vi "Read Coins Config.vi"(8 "error in (no error)":errorcluster) -> (0 "error out":errorcluster, 3 "Value":cluster{"Bolean text":string, "Value":i32}[](array[cluster]))   [LabVIEW 2019, in "Monedas.lvlib"]
uses:
  Monedas.lvlib
  <vilib>/Utility/xml.llb/Read From XML File(string).vi
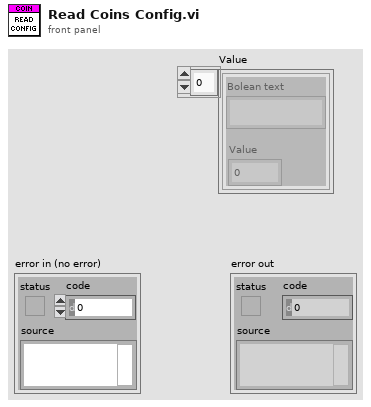
[diagram p1: front panel]
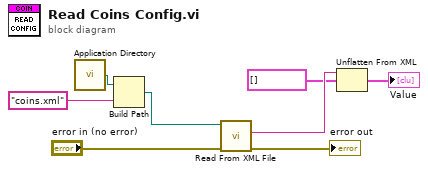
[diagram p0: block diagram]
diagram:
  n1 = call <vilib>:"Application Directory.vi"() -> ("Application Directory"=w8:path)
  n2 = Build Path(base path=w8, name or relative path="coins.xml") -> (appended path=w6:path)
  n3 = call-poly <vilib>:"Read From XML File.vi"("error in (no error)"="error in (no error)", "XML File Path"=w6) -> ("error out"=→"error out":errorcluster, "XML Elements"=w2:string)  [unwired: 7 in, 1 out]
  n4 = Unflatten From XML(xml string=w2, type=cluster{"Bolean text":string, "Value":i32}[] [] ("Coins")) -> (value=→"Value":cluster{"Bolean text":string, "Value":i32}[])  [unwired: 1 in, 1 out]
